vi "Script 2.vi"() -> ()   [LabVIEW 2020]
uses:
  _csmHelper/CSM-Helper.lvclass
  _csmHelper/API/Create From VI Reference.vi
  _csmHelper/API/Destroy.vi
  <vilib>/Utility/miscctls.llb/LVPositionTypeDef.ctl
  <vilib>/Utility/miscctls.llb/LVRectTypeDef.ctl
  _csmHelper/API/Start Undo.vi
  _csmHelper/API/Get CaseFrame Reference By CaseName.vi
  _csmHelper/Properties/Read Block Diagram Ref.vi
  _csmHelper/Properties/Read Case Structure Ref.vi
  _csmHelper/API/Connect StateQ Wire If not Connected.vi
  _csmHelper/API/Stop Undo.vi
  _csmHelper/API/Connect Internal Data Wire If not Connected.vi
  _csmHelper/API/Set Error Tunnel Use Default If not Connected.vi
panel:
  out "Bounds:Area Height 2":u32
  out "Bounds:Area Width 2":u32
  out "Bounds:Area Width":u32
  out "Bounds:Area Height":u32
  in  "element":string="UI: Cursor Set"
  out "index of element":i32[](array[numeric])
  out "Position":T1
  out "output cluster":T1
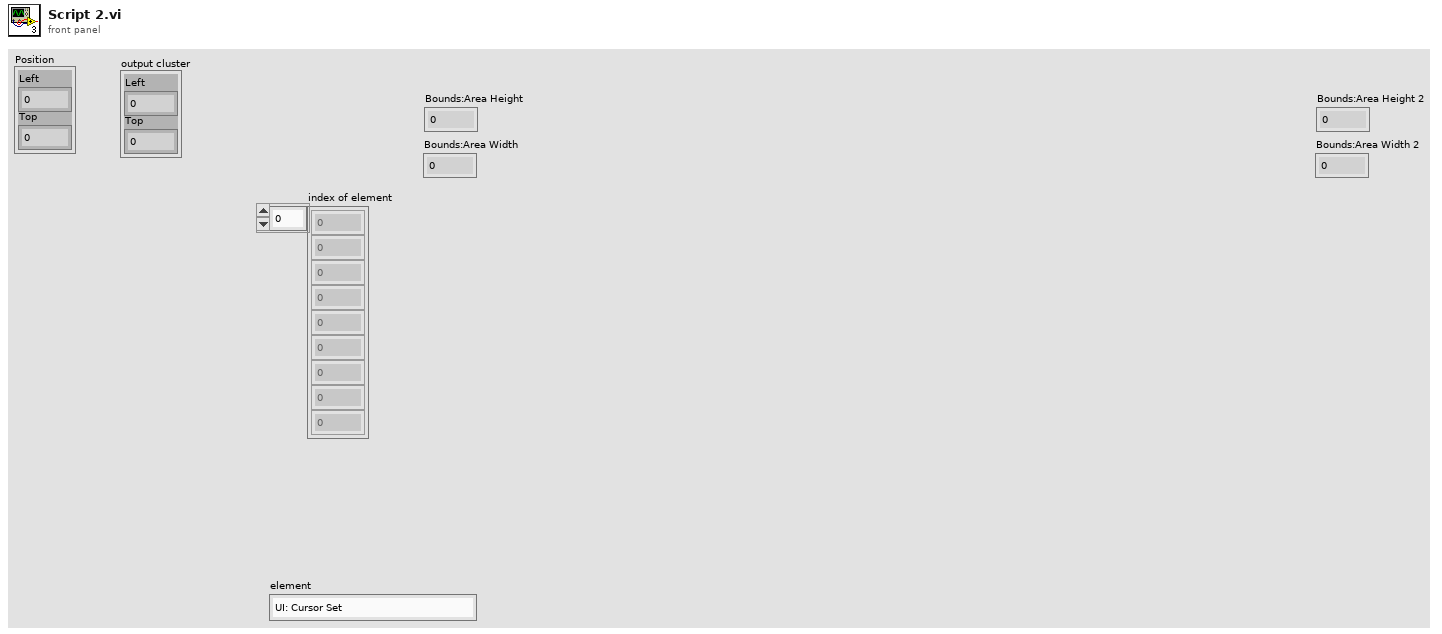
[diagram p1: front panel]
types:
  T1 = typedef "LVPositionTypeDef.ctl" = cluster{"Left":i32, "Top":i32}
  T2 = typedef "LVRectTypeDef.ctl" = cluster{"Left":i16, "Top":i16, "Right":i16, "Bottom":i16}
  T3 = cluster{"InternalData":refnum<vi>, "CSM Name":refnum<vi>, "Last Resp":refnum<vi>, "Remaining State":refnum<vi>, "Arguments":refnum<vi>, "Response Source":refnum<vi>, "Source CSM":refnum<vi>, "Selector":refnum<vi>, "Error":refnum<vi>}
  T4 = cluster{"InternalData":refnum<vi>, "Resp":refnum<vi>, "Remaining State":refnum<vi>, "Error":refnum<vi>}
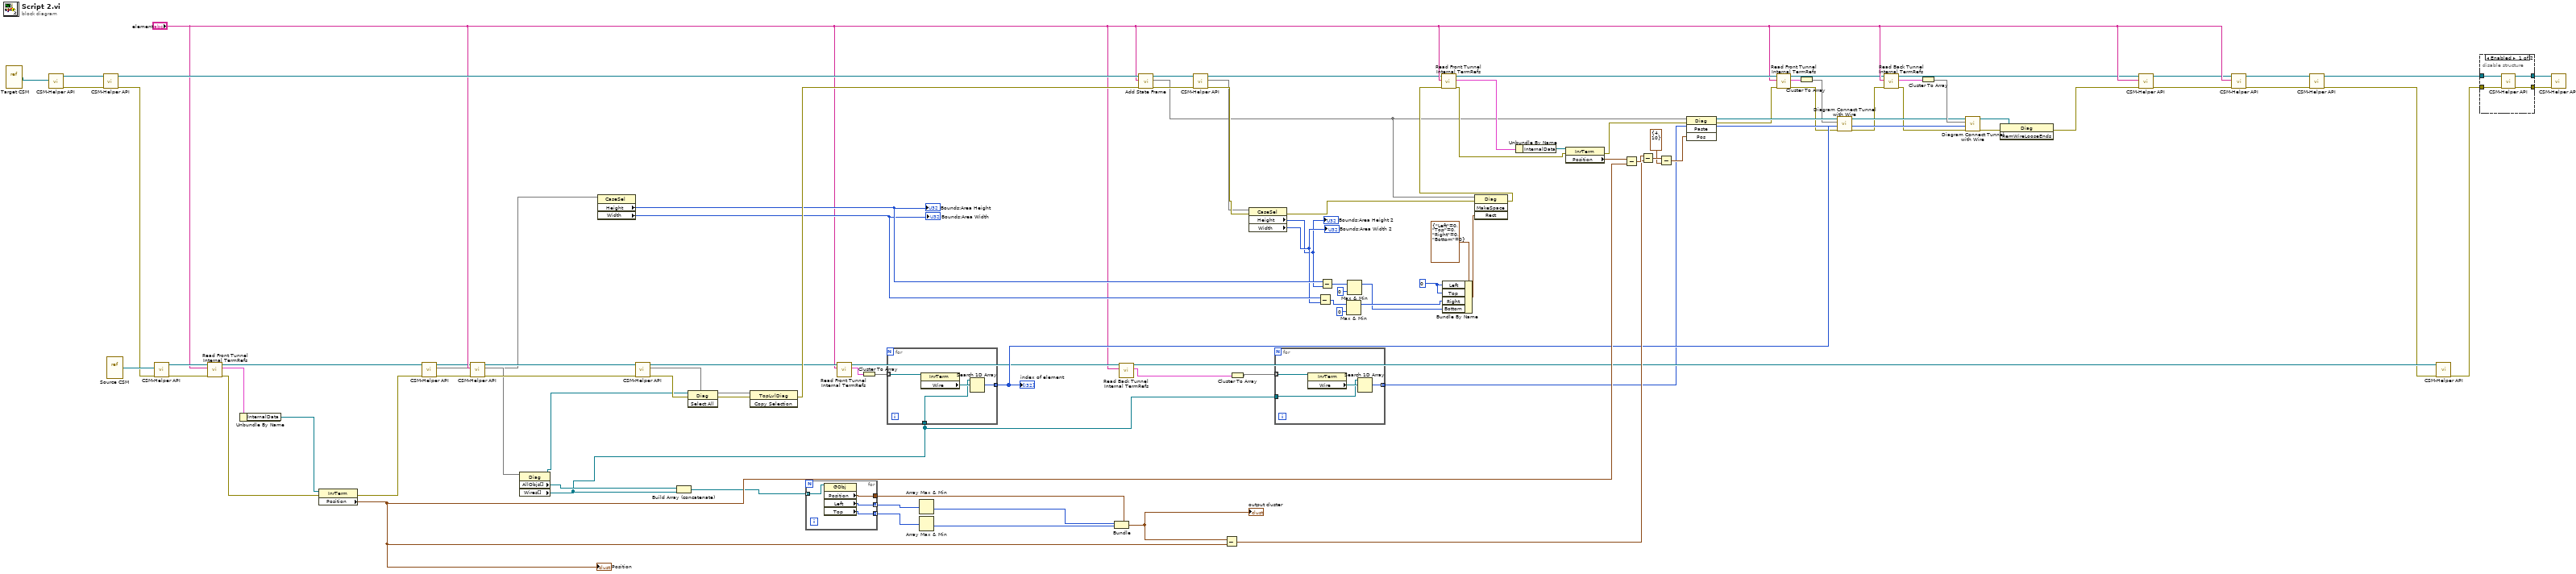
[diagram p0: block diagram]
diagram:
  w18 = i16 0 ("Left")
  n1 = vi-ref "Target CSM.vi"() -> (w96:refnum<vi>)
  n2 = call-poly "CSM-Helper API.vi"("VI"=w96) -> ("error out"=w95:errorcluster, "CSM-Helper.lvclass"=w94:refnum<class "CSM-Helper.lvclass">)  [unwired: 9 in]
  n3 = call-poly "CSM-Helper API.vi"("error in (no error)"=w95, "CSM-Helper in"=w94) -> ("error out"=w69:errorcluster, "CSM-Helper out"=w93:refnum<class "CSM-Helper.lvclass">)  [unwired: 8 in]
  n4 = vi-ref "Source CSM.vi"() -> (w100:refnum<vi>)
  n5 = call-poly "CSM-Helper API.vi"("error in (no error)"=w69, "VI"=w100) -> ("error out"=w83:errorcluster, "CSM-Helper.lvclass"=w84:refnum<class "CSM-Helper.lvclass">)  [unwired: 8 in]
  n6 = call "Read Front Tunnel Internal TermRefs.vi"("error in (no error)"=w83, "case"="element", "CSM-Helper in"=w84) -> ("error out"=w82:errorcluster, "Front Tunnels"=w81:T3, "CSM-Helper out"=w27:refnum<class "CSM-Helper.lvclass">)  [unwired: 6 in]
  n7 = Unbundle By Name(w81) -> ("InternalData"=w80:refnum<vi>)
  n8 = property class="InrTerm"(reference=w80, error in=w82) -> (error out=w28:errorcluster, "Position"=w75:T1)  [unwired: 1 out]
  "Position" <- w75
  n9 = call-poly "CSM-Helper API.vi"("error in (no error)"=w28, "CSM-Helper in"=w27) -> ("error out"=w25:errorcluster, 2:w24, "CSM-Helper out"=w26:refnum<class "CSM-Helper.lvclass">)  [unwired: 6 in, 1 out]
  n10 = call-poly "CSM-Helper API.vi"("error in (no error)"=w25, "CASE"="element", "CSM-Helper in"=w26) -> ("error out"=w99:errorcluster, 2:w44, "CSM-Helper out"=w98:refnum<class "CSM-Helper.lvclass">)  [unwired: 5 in, 1 out]
  n11 = property class="Diag"(reference=w44) -> (reference out=w46:refnum<vi>, "AllObjs[]"=w97:refnum<vi>[], "Wires[]"=w45:refnum<vi>[])  [unwired: 1 in, 1 out]
  n12 = property class="CaseSel"(reference=w24) -> ("Height"=w43:u32, "Width"=w42:u32)  [unwired: 1 in, 2 out]
  "Bounds:Area Height" <- w43
  "Bounds:Area Width" <- w42
  n13 = call-poly "CSM-Helper API.vi"("error in (no error)"=w99, "CSM-Helper in"=w98) -> ("error out"=w67:errorcluster, 2:w63, "CSM-Helper out"=w54:refnum<class "CSM-Helper.lvclass">)  [unwired: 6 in, 1 out]
  n14 = Build Array (concatenate)(w97, w45) -> (w62:refnum<vi>[])
  n15 = invoke class="Diag" method="Select All"(reference=w46, error in=w67) -> (error out=w66:errorcluster)  [unwired: 1 in, 2 out]
  n16 = invoke class="TopLvlDiag" method="Copy Selection"(reference=w63, error in=w66) -> (error out=w68:errorcluster)  [unwired: 1 in, 2 out]
  n17 = for {
    tunnel: w62 -> [w104] mode=indexing
    tunnel: [w103] -> w88 mode=indexing
    tunnel: [w102] -> w89 mode=indexing
    tunnel: [w101] -> w87
    n18 = property class="GObj"(reference=w104) -> ("Position"=w101:T1, "Left"=w103:i32, "Top"=w102:i32)  [unwired: 1 in, 2 out]
  }
  n19 = call "Read Front Tunnel Internal TermRefs.vi"("case"="element", "CSM-Helper in"=w54) -> ("Front Tunnels"=w60:T3, "CSM-Helper out"=w53:refnum<class "CSM-Helper.lvclass">)  [unwired: 7 in, 1 out]
  n20 = Cluster To Array(cluster=w60) -> (array=w59:refnum<vi>[])
  n21 = for {
    tunnel: w45 -> [w107]
    tunnel: [w106] -> w61 mode=indexing
    tunnel: w59 -> [w105] mode=indexing
    n22 = property class="InrTerm"(reference=w105) -> ("Wire"=w108:refnum<vi>)  [unwired: 1 in, 2 out]
    n23 = Search 1D Array(1D array=w107, element=w108) -> (index of element=w106:i32)  [unwired: 1 in]
  }
  "index of element" <- w61
  n24 = Array Max & Min(array=w88) -> (min value=w86:i32)  [unwired: 3 out]
  n25 = Array Max & Min(array=w89) -> (min value=w85:i32)  [unwired: 3 out]
  n26 = Bundle(cluster=w87, "Left"=w86, "Top"=w85) -> (w76:T1)
  "output cluster" <- w76
  n27 = call "Read Back Tunnel Internal TermRefs.vi"("element"="element", "CSM-Helper in"=w53) -> ("Front Tunnels"=w50:T4, "CSM-Helper out"=w52:refnum<class "CSM-Helper.lvclass">)  [unwired: 7 in, 1 out]
  n28 = call "Add State Frame.vi"("error in (no error)"=w68, "element"="element", "CSM-Helper in"=w93) -> ("error out"=w22:errorcluster, 2:w19, "CSM-Helper out"=w70:refnum<class "CSM-Helper.lvclass">)  [unwired: 5 in, 1 out]
  n29 = call-poly "CSM-Helper API.vi"("error in (no error)"=w22, "CSM-Helper in"=w70) -> ("error out"=w21:errorcluster, 2:w20, "CSM-Helper out"=w23:refnum<class "CSM-Helper.lvclass">)  [unwired: 6 in, 1 out]
  n30 = Subtract(x=w76, y=w75) -> (x-y=w73:T1)
  n31 = Cluster To Array(cluster=w50) -> (array=w51:refnum<vi>[])
  n32 = property class="CaseSel"(reference=w20, error in=w21) -> (error out=w29:errorcluster, "Height"=w34:u32, "Width"=w35:u32)  [unwired: 1 out]
  "Bounds:Area Height 2" <- w34
  "Bounds:Area Width 2" <- w35
  n33 = for {
    tunnel: w45 -> [w111]
    tunnel: [w110] -> w49 mode=indexing
    tunnel: w51 -> [w109] mode=indexing
    n34 = property class="InrTerm"(reference=w109) -> ("Wire"=w112:refnum<vi>)  [unwired: 1 in, 2 out]
    n35 = Search 1D Array(1D array=w111, element=w112) -> (index of element=w110:i32)  [unwired: 1 in]
  }
  n36 = Subtract(x=w42, y=w35) -> (x-y=w37:u32)
  n37 = Subtract(x=w43, y=w34) -> (x-y=w40:u32)
  n38 = Max & Min(x=w37, y=u32 0) -> (max(x,y)=w33:u32)  [unwired: 1 out]
  n39 = Max & Min(x=w40, y=u32 0) -> (max(x,y)=w32:u32)  [unwired: 1 out]
  n40 = Bundle By Name(cluster=T2 {"Left"=0, "Top"=0, "Right"=0, "Bottom"=0} ("Rect"), "Left"=w18, "Top"=w18, "Right"=w33, "Bottom"=w32) -> (w36:T2)
  n41 = invoke class="Diag" method="MakeSpace"(reference=w19, error in=w29, "Rect"=w36) -> (error out=w30:errorcluster)  [unwired: 1 in, 3 out]
  n42 = call "Read Front Tunnel Internal TermRefs.vi"("error in (no error)"=w30, "case"="element", "CSM-Helper in"=w23) -> ("error out"=w64:errorcluster, "Front Tunnels"=w58:T3, "CSM-Helper out"=w56:refnum<class "CSM-Helper.lvclass">)  [unwired: 6 in]
  n43 = Unbundle By Name(w58) -> ("InternalData"=w79:refnum<vi>)
  n44 = property class="InrTerm"(reference=w79, error in=w64) -> (error out=w65:errorcluster, "Position"=w78:T1)  [unwired: 1 out]
  n45 = Subtract(x=w78, y=w75) -> (x-y=w77:T1)
  n46 = Subtract(x=w77, y=w73) -> (x-y=w74:T1)
  n47 = Subtract(x=w74, y=T1 {"Left"=4, "Top"=10}) -> (x-y=w72:T1)
  n48 = invoke class="Diag" method="Paste"(reference=w19, error in=w65, "Pos"=w72) -> (reference out=w57:refnum<vi>, error out=w55:errorcluster)  [unwired: 1 in, 2 out]
  n49 = call "Read Front Tunnel Internal TermRefs.vi"("error in (no error)"=w55, "case"="element", "CSM-Helper in"=w56) -> ("error out"=w16:errorcluster, "Front Tunnels"=w15:T3, "CSM-Helper out"=w13:refnum<class "CSM-Helper.lvclass">)  [unwired: 6 in]
  n50 = Cluster To Array(cluster=w15) -> (array=w17:refnum<vi>[])
  n51 = call "Diagram Connect Tunnel with Wire.vi"("error in (no error)"=w16, "FrontEnd Connected Info"=w61, "Front Tunnels"=w17, "Diagram in"=w57) -> ("error out"=w6:errorcluster, "Diagram out"=w8:refnum<vi>)  [unwired: 5 in, 1 out]
  n52 = call "Read Back Tunnel Internal TermRefs.vi"("error in (no error)"=w6, "element"="element", "CSM-Helper in"=w13) -> ("error out"=w5:errorcluster, "Front Tunnels"=w14:T4, "CSM-Helper out"=w12:refnum<class "CSM-Helper.lvclass">)  [unwired: 6 in]
  n53 = Cluster To Array(cluster=w14) -> (array=w9:refnum<vi>[])
  n54 = call "Diagram Connect Tunnel with Wire.vi"("error in (no error)"=w5, "FrontEnd Connected Info"=w49, "Front Tunnels"=w9, "Diagram in"=w8) -> ("error out"=w7:errorcluster, "Diagram out"=w1:refnum<vi>)  [unwired: 5 in, 1 out]
  n55 = invoke class="Diag" method="RemWireLooseEnds"(reference=w1, error in=w7) -> (error out=w2:errorcluster)  [unwired: 1 in, 2 out]
  n56 = call-poly "CSM-Helper API.vi"("error in (no error)"=w2, "case"="element", "CSM-Helper in"=w12) -> ("error out"=w11:errorcluster, "CSM-Helper out"=w10:refnum<class "CSM-Helper.lvclass">)  [unwired: 7 in]
  n57 = call-poly "CSM-Helper API.vi"("error in (no error)"=w11, "case"="element", "CSM-Helper in"=w10) -> ("error out"=w3:errorcluster, "CSM-Helper out"=w4:refnum<class "CSM-Helper.lvclass">)  [unwired: 7 in]
  n58 = call-poly "CSM-Helper API.vi"("error in (no error)"=w3, "CSM-Helper in"=w4) -> ("error out"=w47:errorcluster, "CSM-Helper out"=w48:refnum<class "CSM-Helper.lvclass">)  [unwired: 8 in]
  n59 = call-poly "CSM-Helper API.vi"("error in (no error)"=w47, "CSM-Helper in"=w52) -> ("error out"=w91:errorcluster)  [unwired: 8 in, 1 out]
  n60 = disable-structure shown="Enabled" {
    disable-tunnel: [w116 w118] -> w92
    disable-tunnel: w91 -> [w115 w117]
    disable-tunnel: [w114 w117] -> w90
    disable-tunnel: w48 -> [w113 w118]
    frame Enabled {
      n61 = call-poly "CSM-Helper API.vi"("error in (no error)"=w115, "CSM-Helper in"=w113) -> ("error out"=w114:errorcluster, "CSM-Helper out"=w116:refnum<class "CSM-Helper.lvclass">)  [unwired: 8 in]
    }
    frame Disabled {
    }
  }
  n62 = call-poly "CSM-Helper API.vi"("error in (no error)"=w90, "CSM-Helper in"=w92) -> ()  [unwired: 8 in, 2 out]
